vi "global_receive.vi"() -> ()   [LabVIEW 2025]
panel:
  out "Refresh":bool
  in  "Set Position":dbl[](array[numeric])
  in  "Current Position":dbl[](array[numeric])
  out "Accept Token":string
  in  "Raw Received Message":string
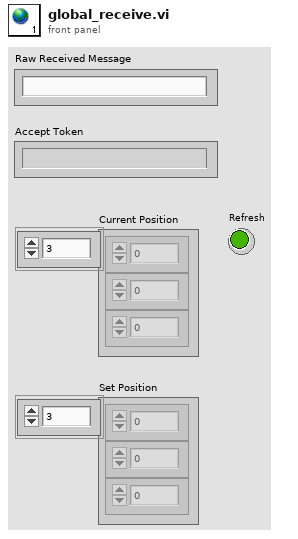
[diagram p1: front panel]
diagram:
